vi "Read_Txt_EEG_File.vi"(7 "SampleRateHz":dbl, 8 "error in (no error)":errorcluster, 9 "ProgressBarRef":refnum<vi>, 10 "ChannelsNum":i32, 11 "EEG file Path in":path) -> (0 "error out":errorcluster, 1 "Events out":T1[](array[typedef]), 2 "ChannelNames out":string[](array[string]), 3 "EEG Refnum out":refnum<data-value>)   [LabVIEW 2016, in "Save Txt To Xml.lvlib"]
uses:
  Trial_Info.ctl
  <vilib>/Utility/file.llb/Read Delimited Spreadsheet (string).vi
  <vilib>/Utility/file.llb/Read Delimited Spreadsheet (DBL).vi
  Save Txt To Xml.lvlib
panel:
  # "This VI is a part of BCI Design library, http://www.ru-bci.org \nCopyright © 2020, Sotnikov Peter, All rights reserved. License: GNU GPLv3"
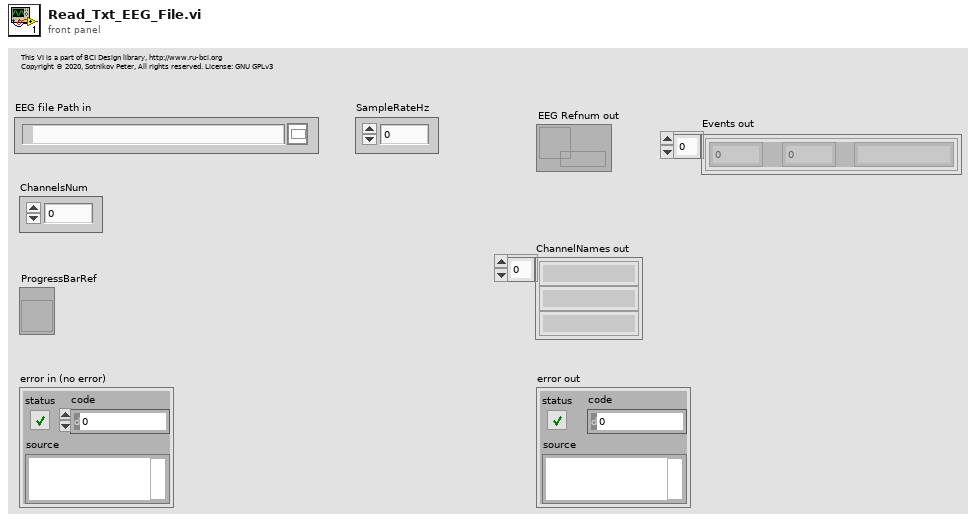
[diagram p1: front panel]
types:
  T1 = typedef "Save Txt To Xml.lvlib/Trial_Info.ctl" = cluster{"Start Position":i32, "End Position":i32, "Class":string}
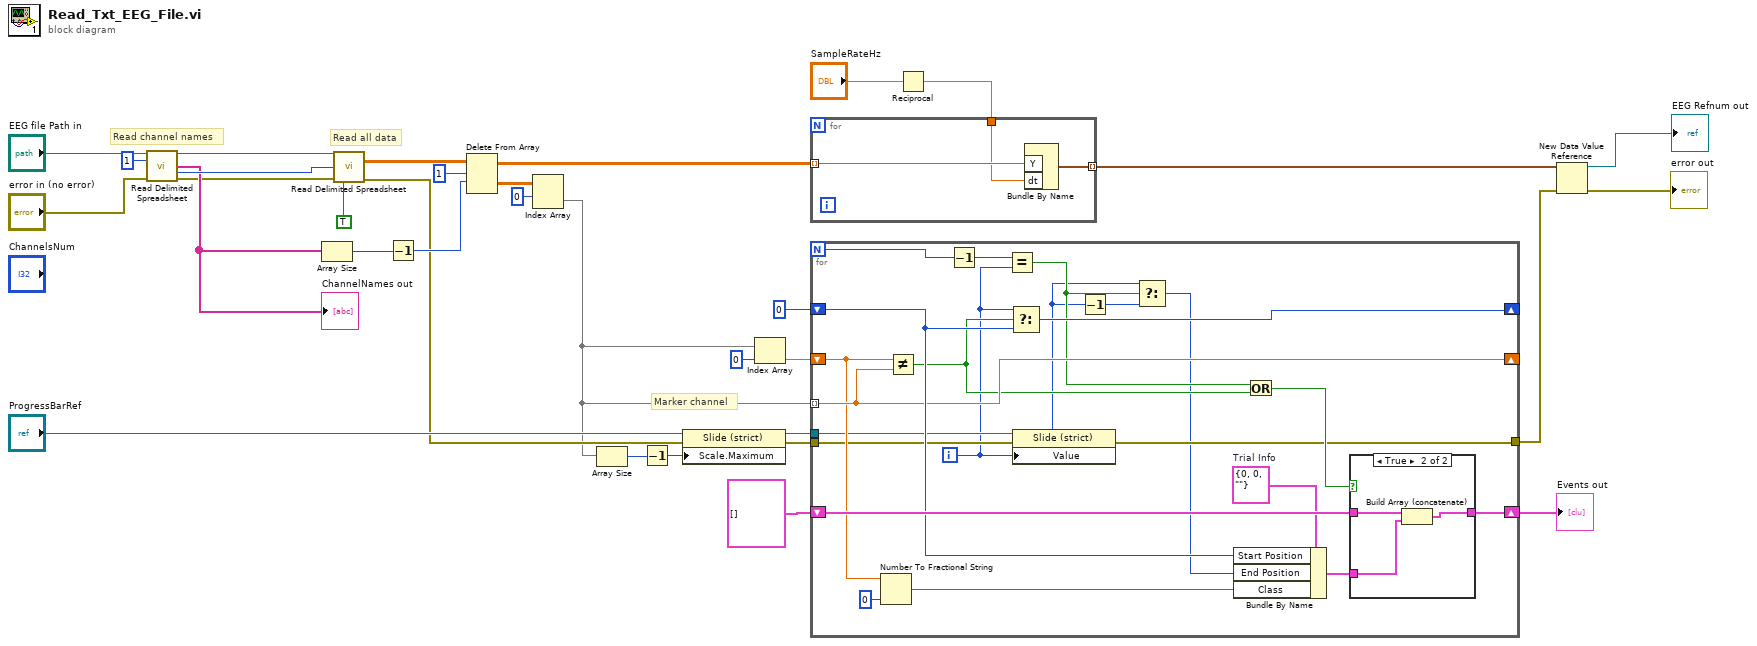
[diagram p0: block diagram]
diagram:
  # "Marker channel"
  # "Read channel names"
  # "Read all data"
  n1 = call-poly <vilib>:"Read Delimited Spreadsheet.vi"("file path (dialog if empty)"="EEG file Path in", "number of rows (all:-1)"=1, "error in (no error)"="error in (no error)") -> ("new file path (Not A Path if cancelled)"=w27:path, "first row"=w24:string[], "mark after read (chars.)"=w26:i32, "error out"=w10:errorcluster)  [unwired: 7 in, 2 out]
  "ChannelNames out" <- w24
  n2 = Array Size(array=w24) -> (size(s)=w23:i32)
  n3 = call-poly <vilib>:"Read Delimited Spreadsheet.vi"("file path (dialog if empty)"=w27, "start of read offset (chars.:0)"=w26, "error in (no error)"=w10, "transpose? (F)"=TRUE) -> ("all rows"=w22:dbl[][], "error out"=w9:errorcluster)  [unwired: 6 in, 4 out]
  n4 = Decrement(x=w23) -> (x-1=w21:i32)
  n5 = Delete From Array(array=w22, length=1, index (row)=w21) -> (deleted portion=w14:dbl[][], array with subset deleted=w19:dbl[][])  [unwired: 1 in]
  n6 = Index Array(array=w14, index (row)=0) -> (element=w7:dbl[])  [unwired: 1 in]
  n7 = Array Size(array=w7) -> (size(s)=w2:i32)
  n8 = Decrement(x=w2) -> (x-1=w1:i32)
  n9 = property class="Slide (strict)"(reference="ProgressBarRef", error in=w9, "Scale.Maximum"=w1) -> (reference out=w6:refnum<vi>, error out=w4:errorcluster)
  n10 = Index Array(array=w7, index=0) -> (element=w15:dbl)
  n11 = for {
    N -> [w46]
    tunnel: w7 -> [w49] mode=indexing
    shift-right: [w52] -> w5
    shift-left: T1[] [] -> [w53]
    shift-right: [w49] -> _
    shift-left: w15 -> [w48]
    shift-right: [w54] -> _
    shift-left: 0 -> [w50]
    tunnel: w6 -> [w41]
    tunnel: w4 -> [w39]
    tunnel: [w38] -> w3
    i -> [w35]
    w40 = T1 {"Start Position"=0, "End Position"=0, "Class"=""}  # Trial Info
    n12 = Number To Fractional String(number=w48, precision (6)=i16 0) -> (F-format string=w47:string)  [unwired: 2 in]
    n13 = Not Equal?(x=w48, y=w49) -> (x != y?=w44:bool)
    n14 = Decrement(x=w46) -> (x-1=w45:i32)
    n15 = Equal?(x=w45, y=w35) -> (x = y?=w37:bool)
    n16 = Select(t=w35, s=w44, f=w50) -> (s? t:f=w54:i32)
    n17 = property class="Slide (strict)"(reference=w41, error in=w39, "Value"=w35) -> (error out=w38:errorcluster)  [unwired: 1 out]
    n18 = Decrement(x=w35) -> (x-1=w36:i32)
    n19 = Select(t=w35, s=w37, f=w36) -> (s? t:f=w34:i32)
    n20 = Bundle By Name(cluster=w40, "Start Position"=w50, "End Position"=w34, "Class"=w47) -> (w51:T1)
    n21 = Or(x=w37, y=w44) -> (x .or. y?=w43:bool)
    n22 = case shown="True" w43 {
      tunnel: w53 -> [w55 w58]
      tunnel: [w55 w56] -> w52
      tunnel: w51 -> [_ w57]
      frame False {
      }
      frame True {
        n23 = Build Array (concatenate)(w58, w57) -> (w56:T1[])
      }
    }
  }
  "Events out" <- w5
  n24 = Reciprocal(x="SampleRateHz") -> (1/x=w18:dbl)
  n25 = for {
    tunnel: w19 -> [w61] mode=indexing
    tunnel: w18 -> [w60]
    tunnel: [w59] -> w17 mode=indexing
    n26 = Bundle By Name("Y"=w61, "dt"=w60) -> (w59:waveform(dbl))  [unwired: 1 in]
  }
  n27 = New Data Value Reference(data value=w17, error in=w3) -> (data value reference=→"EEG Refnum out":refnum<data-value>, error out=→"error out":errorcluster)
